vi "HoloPy_test_typr_var.vi"(8 "error in (no error)":errorcluster, 9 "VAR":u32, 10 "Application Directory":path, 11 "Refnum in":refnum<k35>) -> (0 "error out":errorcluster, 2 "return value":string, 3 "Refnum out":refnum<k35>)   [LabVIEW 2023, in "holoTracker.lvlib"]
uses:
  holoTracker.lvlib
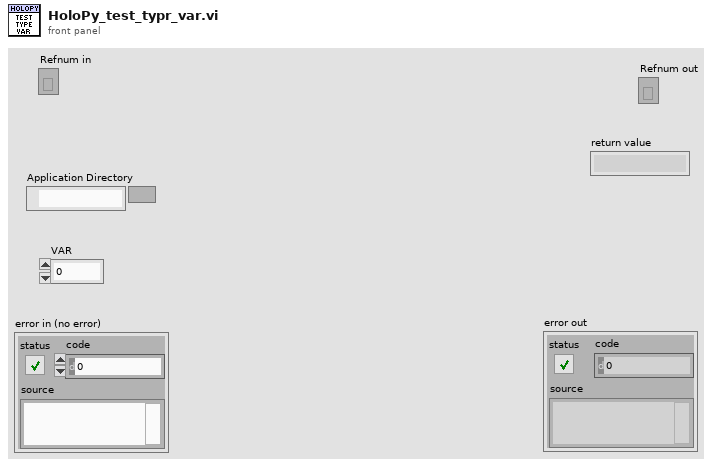
[diagram p1: front panel]
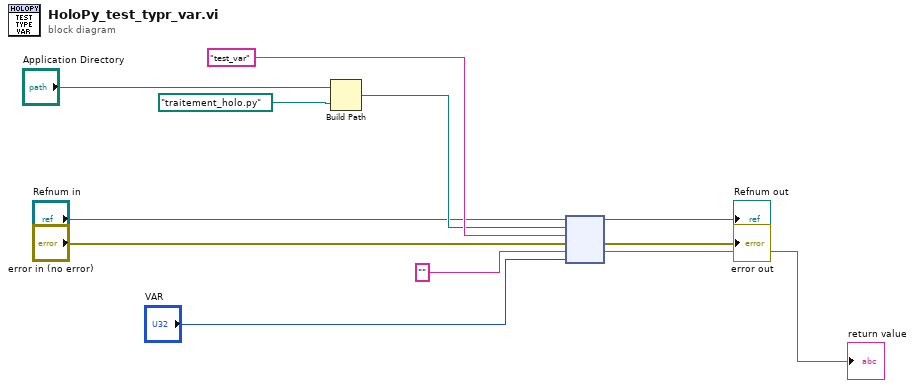
[diagram p0: block diagram]
diagram:
  n1 = Build Path(base path="Application Directory", name or relative path=path "traitement_holo.py") -> (appended path=w10:path)
  n2 = node("Refnum in", w10, "test_var" ("function name"), "error in (no error)", "", "VAR") -> (→"Refnum out":refnum<k35>, →"error out":errorcluster, →"return value":string)  [unwired: 1 in, 2 out]
